vi "Close imagej files.vi"(2 "File Num":u16) -> ()   [LabVIEW 2015]
uses:
  user32.dll
panel:
  out "concatenated string":string
  out "Error output":errorcluster caption="Error Output"
  in  "Error Input":errorcluster
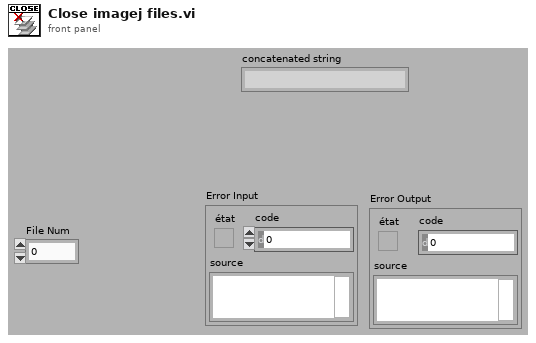
[diagram p1: front panel]
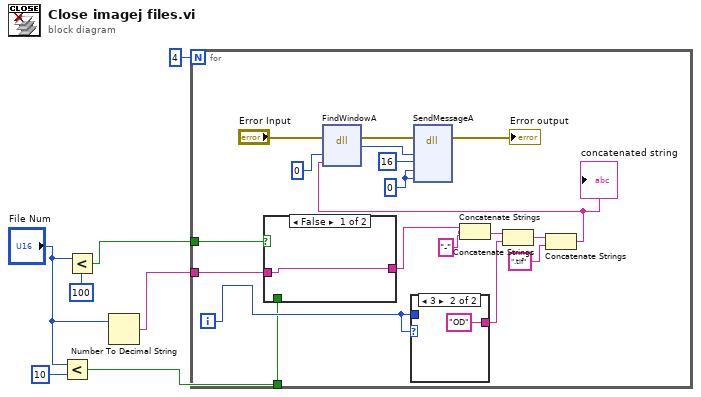
[diagram p0: block diagram]
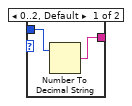
[diagram p2: hidden frame]
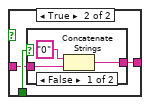
[diagram p3: hidden frame]
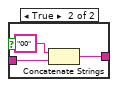
[diagram p4: hidden frame]
diagram:
  n1 = Less?(x="File Num", y=u16 10) -> (x < y?=w4:bool)
  n2 = Less?(x="File Num", y=u16 100) -> (x < y?=w5:bool)
  n3 = Number To Decimal String(number="File Num") -> (decimal integer string=w2:string)  [unwired: 1 in]
  n4 = for {
    N: 4 -> [_]
    tunnel: w5 -> [w17]
    tunnel: w4 -> [w16]
    tunnel: w2 -> [w15]
    i -> [w18]
    w19 = u32 0 ("lParam")
    n5 = case shown="False" w17 {
      tunnel: w16 -> [_ w32]
      tunnel: w15 -> [w29 w31]
      tunnel: [w29 w30] -> w9
      frame False {
      }
      frame True {
        n6 = case shown="False" w32 {
          tunnel: w31 -> [w34 w38]
          tunnel: [w33 w36] -> w30
          frame False {
            n7 = Concatenate Strings("0" ("字符串"), w34) -> (w33:string)
          }
          frame True {
            n8 = Concatenate Strings("00" ("字符串"), w38) -> (w36:string)
          }
        }
      }
    }
    n9 = case shown="3" w18 {
      tunnel: w18 -> [w27 _]
      tunnel: [w26 "OD"] -> w12
      frame 0..2, Default {
        n10 = Number To Decimal String(number=w27) -> (decimal integer string=w26:string)  [unwired: 1 in]
      }
      frame 3 {
      }
    }
    n11 = Concatenate Strings(w9, "-" ("字符串")) -> (w11:string)
    n12 = Concatenate Strings(w11, w12) -> (w13:string)
    n13 = Concatenate Strings(w13, ".tif" ("字符串")) -> (w8:string)
    "concatenated string" <- w8
    n14 = dll-call lib="user32.dll" fn="FindWindowA" label="FindWindow"(error in="Error Input", "lpszClassName"=0, "lpszWindowName"=w8) -> (error out=w22:errorcluster, "hWnd"=w21:u32)  [unwired: 4 in, 1 out]
    n15 = dll-call lib="user32.dll" fn="SendMessageA" label="SendMessage"(error in=w22, "hWnd"=w21, "uMsg"=u32 16, "wParam"=w19, "lParam"=w19) -> (error out=→"Error output":errorcluster)  [unwired: 7 in, 1 out]
  }
